vi "load_plot_window_dyn_2.vi"(8 "error in (no error)":errorcluster, 10 "Ext PlotObjQueue in":refnum<queue>, 11 "Plots in":refnum<class "Plots.lvclass">) -> (0 "error out":errorcluster, 3 "Plots out":refnum<class "Plots.lvclass">)   [LabVIEW 2018]
doc: "loads the plot_window.vit dynamically"
uses:
  Classes/Plots/Plots.lvclass
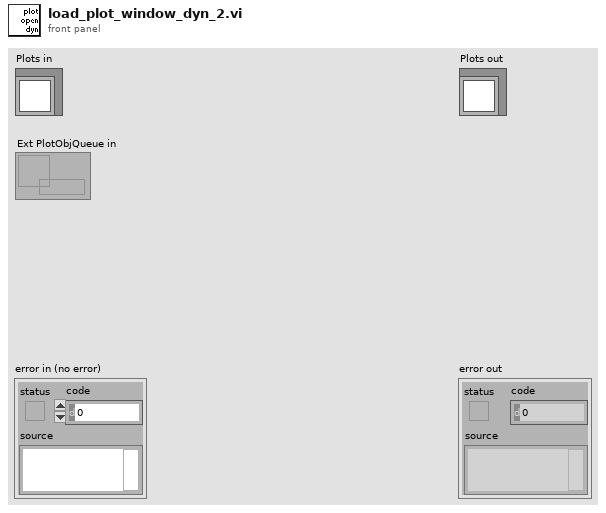
[diagram p1: front panel]
types:
  T1 = enum32{"Invalid", "Standard", "Closed", "Hidden", "Minimized", "Maximized"}
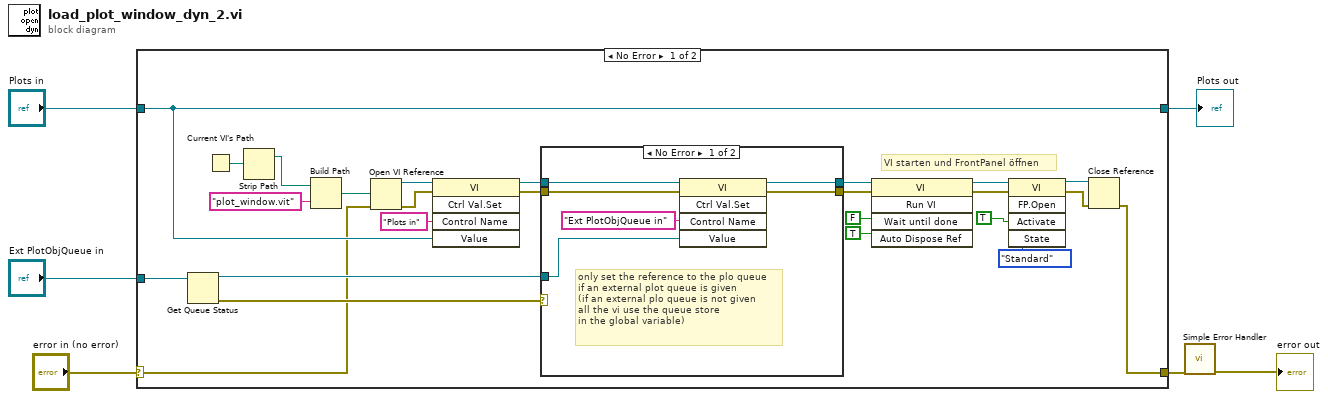
[diagram p0: block diagram]
diagram:
  n1 = case shown="No Error" "error in (no error)" {
    selector: "error in (no error)" -> [w8 w41]
    tunnel: [w7 w41] -> w2
    tunnel: [w17 w40] -> w4
    tunnel: "Plots in" -> [w17 w40]
    tunnel: "Ext PlotObjQueue in" -> [w11 _]
    frame No Error {
      # "VI starten und FrontPanel öffnen"
      n2 = Get Queue Status(queue=w11) -> (queue out=w9:refnum<queue>, error out=w10:errorcluster)  [unwired: 2 in, 6 out]
      n3 = Current VI's Path() -> (path=w28:path)
      n4 = Strip Path(path=w28) -> (stripped path=w29:path)  [unwired: 1 out]
      n5 = Build Path(base path=w29, name or relative path="plot_window.vit") -> (appended path=w16:path)
      n6 = Open VI Reference(vi path=w16, error in (no error)=w8) -> (vi reference=w30:refnum<vi>, error out=w31:errorcluster)  [unwired: 4 in]
      n7 = invoke class="VI" method="Ctrl Val.Set"(reference=w30, error in=w31, "Control Name"="Plots in", "Value"=w17) -> (reference out=w15:refnum<vi>, error out=w14:errorcluster)  [unwired: 1 in, 3 out]
      n8 = case shown="No Error" w10 {
        tunnel: w15 -> [w37 w39]
        tunnel: w14 -> [w36 w38]
        tunnel: [w35 w39] -> w13
        tunnel: [w34 w38] -> w12
        tunnel: w9 -> [w32 _]
        frame No Error {
          # "only set the reference to the plo queue\nif an external plot queue is given\n(if an external plo queue is not given\nall the vi use the queue store\nin the global variable)"
          n9 = invoke class="VI" method="Ctrl Val.Set"(reference=w37, error in=w36, "Control Name"="Ext PlotObjQueue in", "Value"=w32) -> (reference out=w35:refnum<vi>, error out=w34:errorcluster)  [unwired: 1 in, 3 out]
        }
        frame Error {
        }
      }
      n10 = invoke class="VI" method="Run VI"(reference=w13, error in=w12, "Wait until done"=FALSE, "Auto Dispose Ref"=TRUE) -> (reference out=w20:refnum<vi>, error out=w21:errorcluster)  [unwired: 1 in, 3 out]
      n11 = invoke class="VI" method="FP.Open"(reference=w20, error in=w21, "Activate"=TRUE, "State"=T1."Standard") -> (reference out=w24:refnum<vi>, error out=w25:errorcluster)  [unwired: 1 in, 3 out]
      n12 = Close Reference(reference=w24, error in (no error)=w25) -> (error out=w7:errorcluster)
    }
    frame Error {
    }
  }
  "Plots out" <- w4
  n13 = call <vilib>:"Simple Error Handler.vi"("error in (no error)"=w2) -> ("error out"=→"error out":errorcluster)  [unwired: 4 in, 4 out]
